vi "upLoadFile.vi"(10 "file path (dialog if empty)":path) -> (0 "time_B_noInter":dbl[](array[numeric]) format="%.2f", 1 "VE_B_noInter":dbl[](array[numeric]), 2 "time_E_noInter":dbl[](array[numeric]) format="%.2f", 3 "VE_E_noInter":dbl[](array[numeric]), 4 "time_E":dbl[](array[numeric]) format="%.2f", 5 "time_B":dbl[](array[numeric]) format="%.2f", 6 "VE_E":dbl[](array[numeric]), 7 "VE_B":dbl[](array[numeric]))   [LabVIEW 2012]
uses:
  <vilib>/Utility/file.llb/Read From Spreadsheet File (string).vi
panel:
  out "B":i32
  out "E":i32
  out "R":i32
  out "finalSize":i32
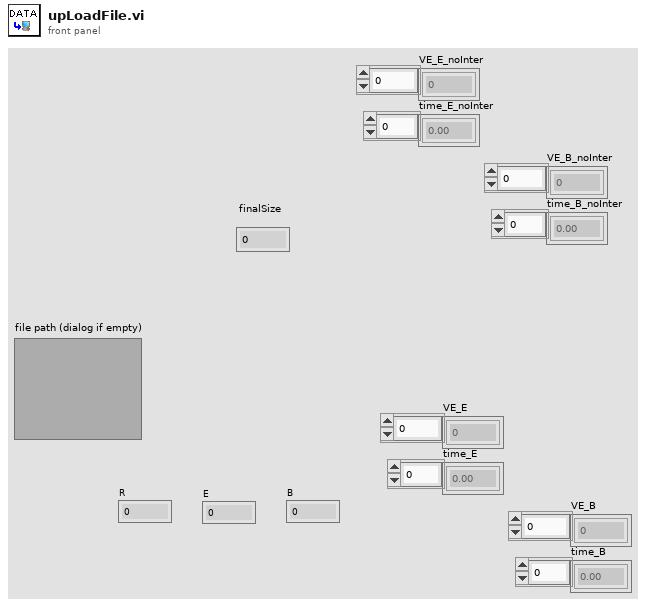
[diagram p1: front panel]
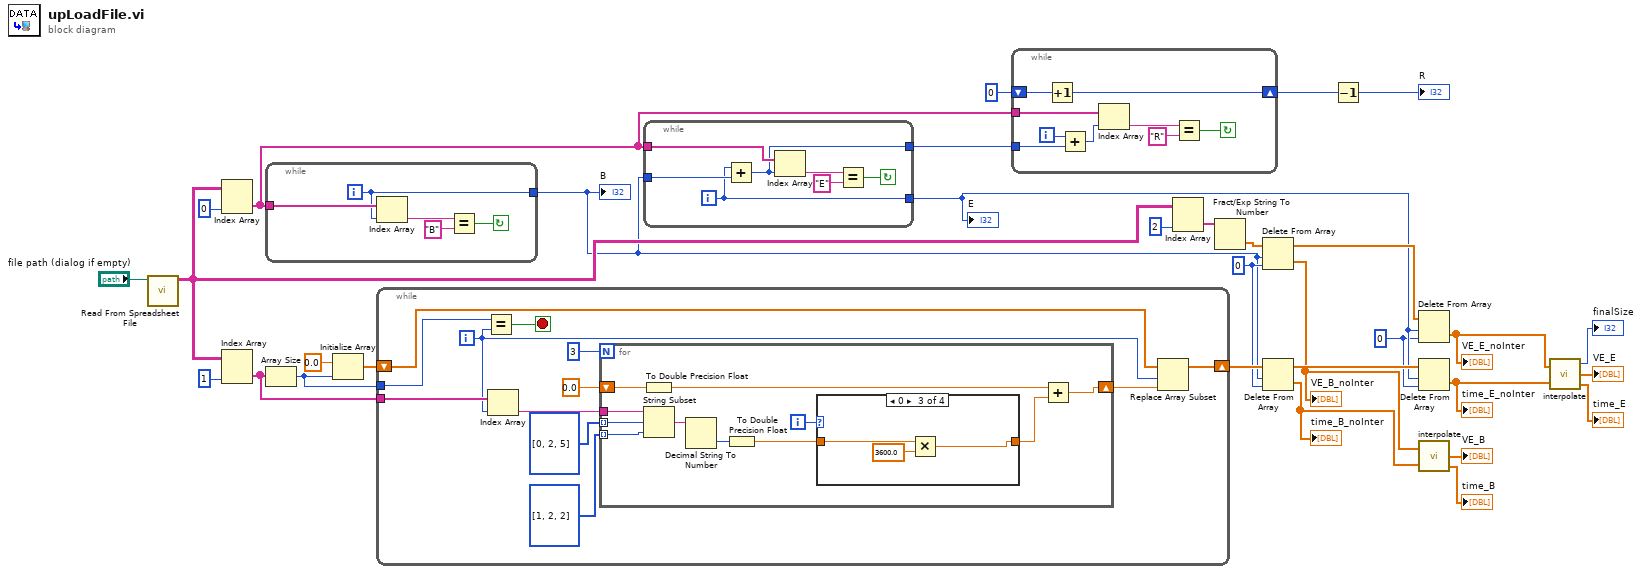
[diagram p0: block diagram]
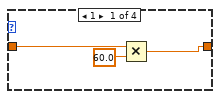
[diagram p2: hidden frame]
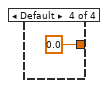
[diagram p4: hidden frame]
diagram:
  w10 = 0 ("index")
  w15 = 0 ("index")
  n1 = call-poly <vilib>:"Read From Spreadsheet File.vi"("file path (dialog if empty)"="file path (dialog if empty)") -> ("all rows"=w25:string[][])  [unwired: 6 in, 4 out]
  n2 = Index Array(array=w25, index (col)=0 ("disabled index (col)")) -> (element=w22:string[])  [unwired: 1 in]
  n3 = Index Array(array=w25, index (col)=1 ("disabled index (col)")) -> (element=w28:string[])  [unwired: 1 in]
  n4 = while {
    tunnel: w22 -> [w37]
    tunnel: [w33] -> w14
    i -> [w33]
    stop <- w34 continue-if-true
    n5 = Index Array(array=w37, index=w33) -> (element=w36:string)
    n6 = Equal?(x=w36, y="B") -> (x = y?=w34:bool)
  }
  "B" <- w14
  n7 = Array Size(array=w28) -> (size(s)=w17:i32)
  n8 = Initialize Array(0.0, w17) -> (w27:dbl[])
  n9 = while {
    tunnel: w28 -> [w47]
    tunnel: w17 -> [w49]
    shift-right: [w45] -> w18
    shift-left: w27 -> [w46]
    i -> [w44]
    stop <- w48 stop-if-true
    n10 = Equal?(x=w49, y=w44) -> (x = y?=w48:bool)
    n11 = Index Array(array=w47, index=w44) -> (element=w43:string)
    n12 = for {
      N: 3 -> [_]
      tunnel: w43 -> [w56]
      tunnel: i32[] [0, 2, 5] -> [w55] mode=indexing
      shift-right: [w50] -> w39
      shift-left: 0.0 -> [w58]
      tunnel: i32[] [1, 2, 2] -> [w54] mode=indexing
      i -> [w60]
      n13 = To Double Precision Float(number=w58) -> (double precision float=w57:dbl)
      n14 = String Subset(string=w56, offset (0)=w55, length (rest)=w54) -> (substring=w53:string)
      n15 = Decimal String To Number(string=w53) -> (number=w52:i32)  [unwired: 2 in, 1 out]
      n16 = To Double Precision Float(number=w52) -> (double precision float=w51:dbl)
      n17 = case shown="0" w60 {
        tunnel: [w62 w64 w66 0.0] -> w59
        tunnel: w51 -> [w61 w64 w65 _]
        frame 1 {
          n18 = Multiply(x=w61, y=60.0) -> (x*y=w62:dbl)
        }
        frame 2 {
        }
        frame 0 {
          n19 = Multiply(x=w65, y=3600.0) -> (x*y=w66:dbl)
        }
        frame Default {
        }
      }
      n20 = Add(x=w57, y=w59) -> (x+y=w50:dbl)
    }
    n21 = Replace Array Subset(array=w46, new element=w39, index=w44) -> (w45:dbl[])
  }
  n22 = while {
    tunnel: w22 -> [w75]
    tunnel: w14 -> [w71]
    tunnel: [w70] -> w11
    tunnel: [w69] -> w20
    i -> [w70]
    stop <- w72 continue-if-true
    n23 = Add(x=w70, y=w71) -> (x+y=w69:i32)
    n24 = Index Array(array=w75, index=w69) -> (element=w74:string)
    n25 = Equal?(x=w74, y="E") -> (x = y?=w72:bool)
  }
  "E" <- w11
  n26 = while {
    tunnel: w22 -> [w82]
    shift-right: [w84] -> w21
    shift-left: 0 -> [w83]
    tunnel: w20 -> [w76]
    i -> [w81]
    stop <- w78 continue-if-true
    n27 = Increment(x=w83) -> (x+1=w84:i32)
    n28 = Add(x=w81, y=w76) -> (x+y=w77:i32)
    n29 = Index Array(array=w82, index=w77) -> (element=w80:string)
    n30 = Equal?(x=w80, y="R") -> (x = y?=w78:bool)
  }
  n31 = Index Array(array=w25, index (col)=2) -> (element=w29:string[])  [unwired: 1 in]
  n32 = Fract/Exp String To Number(string=w29) -> (number=w13:dbl[])  [unwired: 3 in, 1 out]
  n33 = Delete From Array(array=w13, length=w14, index=w15) -> (deleted portion=w8:dbl[], array with subset deleted=w12:dbl[])
  "VE_B_noInter" <- w8
  n34 = Delete From Array(array=w18, length=w14, index=w15) -> (deleted portion=w9:dbl[], array with subset deleted=w16:dbl[])
  "time_B_noInter" <- w9
  n35 = Decrement(x=w21) -> (x-1=→"R":i32)
  n36 = Delete From Array(array=w12, length=w11, index=w10) -> (deleted portion=w4:dbl[])  [unwired: 1 out]
  "VE_E_noInter" <- w4
  n37 = Delete From Array(array=w16, length=w11, index=w10) -> (deleted portion=w5:dbl[])  [unwired: 1 out]
  "time_E_noInter" <- w5
  n38 = call "interpolate.vi"("Ve_in"=w8, "time_in"=w9) -> ("Ve_out"=→"VE_B":dbl[], "time_out"=→"time_B":dbl[])  [unwired: 1 out]
  n39 = call "interpolate.vi"("Ve_in"=w4, "time_in"=w5) -> ("finalSize"=→"finalSize":i32, "Ve_out"=→"VE_E":dbl[], "time_out"=→"time_E":dbl[])
